vi "XPath表达式.vi"(7 "添加的路径":path, 11 "XPath expression":string caption="XPath表达式") -> (3 "数组":cluster{string, i32}[](array[cluster]))   [LabVIEW 2016, in "斯坦道总磷.lvlib"]
uses:
  <vilib>/xml/Load XML File.vi
  <vilib>/xml/Close Reference(Node).vi
  <vilib>/xml/NI_XML.lvlib
  D:/Program Files (x86)/National Instruments/LabVIEW 2016/resource/objmgr/DOMUserDefRef.rc
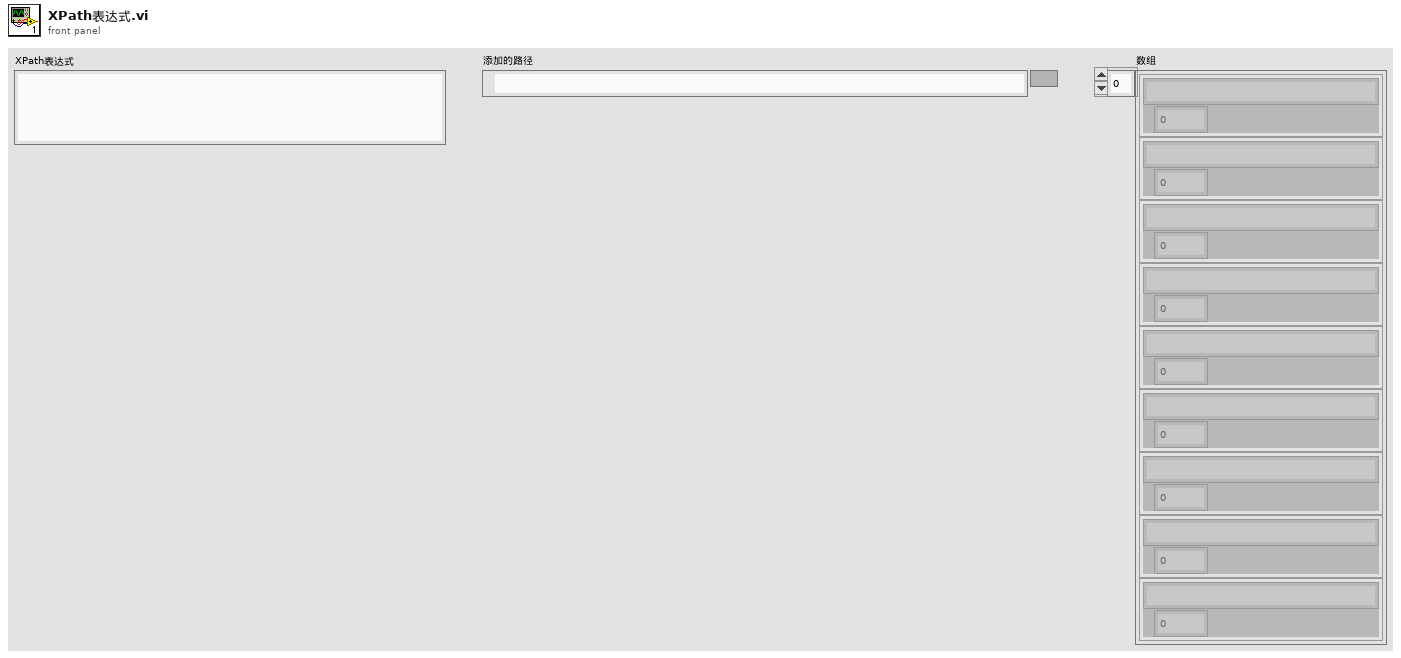
[diagram p1: front panel]
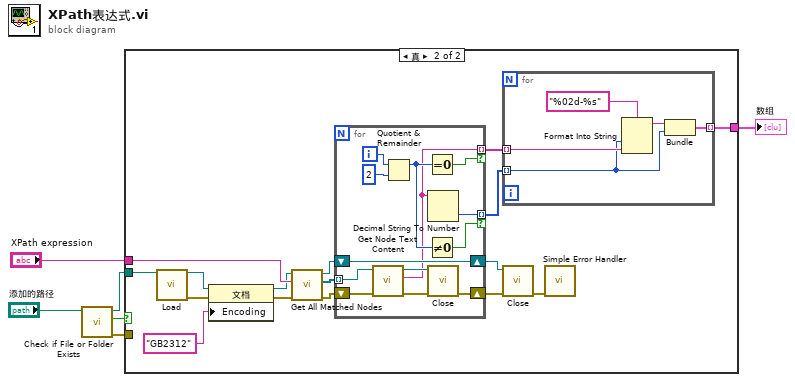
[diagram p0: block diagram]
diagram:
  n1 = call <vilib>:"Check if File or Folder Exists.vi"("path"="添加的路径") -> ("error out"=w1:errorcluster, "file or folder exists?"=w2:bool, "dup path"=w5:path)  [unwired: 8 in]
  n2 = case shown="真" w2 {
    tunnel: w5 -> [_ w22]
    tunnel: "XPath expression" -> [_ w15]
    tunnel: [_ w9] -> w3
    tunnel: w1 -> [_ _]
    frame False {
    }
    frame True {
      n3 = call-poly <vilib>:"Load.vi"("path to XML document"=w22) -> ("DOM document out"=w19:refnum<k20>, "error out"=w18:errorcluster)  [unwired: 12 in, 1 out]
      n4 = property on="属性节点" class="文档"(reference=w19, error in=w18, "Encoding"="GB2312" ("文档编码")) -> (reference out=w13:refnum<k20>, error out=w12:errorcluster)
      n5 = call <vilib>:"Get All Matched Nodes.vi"("error in (no error)"=w12, "XPath expression"=w15, "node in"=w13) -> ("error out"=w16:errorcluster, "node result array"=w17:refnum<k20>[], "node out"=w11:refnum<k20>)  [unwired: 6 in]
      n6 = for {
        tunnel: w17 -> [w36] mode=indexing
        shift-right: [w37] -> w14
        shift-left: w16 -> [w40]
        shift-right: [w35] -> w10
        shift-left: w11 -> [w35]
        tunnel: [w28] -> w8 mode=indexing if=w32
        tunnel: [w29] -> w7 mode=indexing if=w30
        i -> [w34]
        n7 = call <vilib>:"Get Node Text Content.vi"("error in (no error)"=w40, "node in"=w36) -> ("error out"=w38:errorcluster, "node text"=w28:string, "node out"=w39:refnum<k20>)  [unwired: 7 in]
        n8 = Quotient & Remainder(x=w34, y=2) -> (x-y*floor(x/y)=w31:i32)  [unwired: 1 out]
        n9 = Equal To 0?(x=w31) -> (x = 0?=w32:bool)
        n10 = Not Equal To 0?(x=w31) -> (x != 0?=w30:bool)
        n11 = Decimal String To Number(string=w28) -> (number=w29:i32)  [unwired: 2 in, 1 out]
        n12 = call-poly <vilib>:"Close.vi"("error in (no error)"=w38, "node"=w39) -> ("error out"=w37:errorcluster)  [unwired: 7 out]
      }
      n13 = for {
        tunnel: w8 -> [w25] mode=indexing
        tunnel: w7 -> [w23] mode=indexing
        tunnel: [w27] -> w9 mode=indexing
        n14 = Format Into String(format string="%02d-%s" ("格式字符串"), w23, w25) -> (resulting string=w24:string)  [unwired: 2 in, 1 out]
        n15 = Bundle(w24, w23) -> (w27:cluster{string, i32})  [unwired: 1 in]
      }
      n16 = call-poly <vilib>:"Close.vi"("error in (no error)"=w14, "node"=w10) -> ("error out"=w21:errorcluster)  [unwired: 7 out]
      n17 = call <vilib>:"Simple Error Handler.vi"("error in (no error)"=w21) -> ()  [unwired: 4 in, 5 out]
    }
  }
  "数组" <- w3
